vi "BPM.vi"() -> ()   [LabVIEW 2016]
uses:
  <vilib>/rvi/interface/nirviOpenFPGA/nirviOpenFPGA.xnode
  FPGA/BPM FPGA.vi
  <vilib>/rvi/interface/nirviReadWriteControl/nirviReadWriteControl.xnode
  <vilib>/Instr/_visa.llb/VISA Configure Serial Port (Instr).vi
  <vilib>/Utility/error.llb/Error Cluster From Error Code.vi
  <vilib>/rvi/errors/niLvFpgaAdjustHostInterfaceError.vi
  FPGA Bitfiles/Controlsoftware2_FPGATarget7_BPMFPGA_nBaxFvqMFXU.lvbitx
  <vilib>/FPGAPlugInAG/cRIO-9074/niLvFpga_Open_cRIO-9074.vi
  NiFpgaLv.dll
panel:
  out "einzel readbacks setpoints":fxp<+/-,26,5>[](array[numeric])
  out "einzel readbacks readbacks":fxp<+/-,26,5>[](array[numeric])
  out "chop index":i32
  out "element":string="0.00E+00\r\n"
  in  "source cage Ion gauge Cluster 4":T1
  out "source cage Ion gauge Cluster 2":T1={"beam line pressure  Gauge "="9.90E+09\r\n", "Turbo convectorn Gauge "="0.00E+00\r\n", "Steerer Convectro Gauge "="2.40E-08\r\n", "Ion gauge2"="7.60E-01\r\n"}
  out "read buffer":string="0.00E+00\r\n"
  out "error out":errorcluster
  out "BPM 2 x10":bool
  out "BPM 2":bool
  out "BPM 1 x10":bool
  out "BPM 1":bool
  # "0 run\n1 divert\n2 offset\n3 chop to detector"
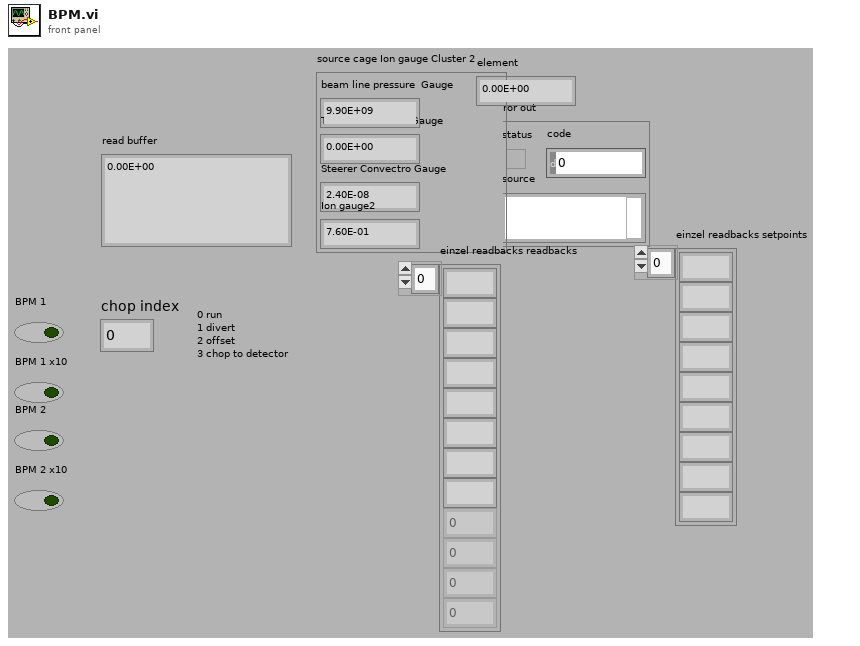
[diagram p1: front panel]
types:
  T1 = cluster{"beam line pressure  Gauge ":string, "Turbo convectorn Gauge ":string, "Steerer Convectro Gauge ":string, "Ion gauge2":string}
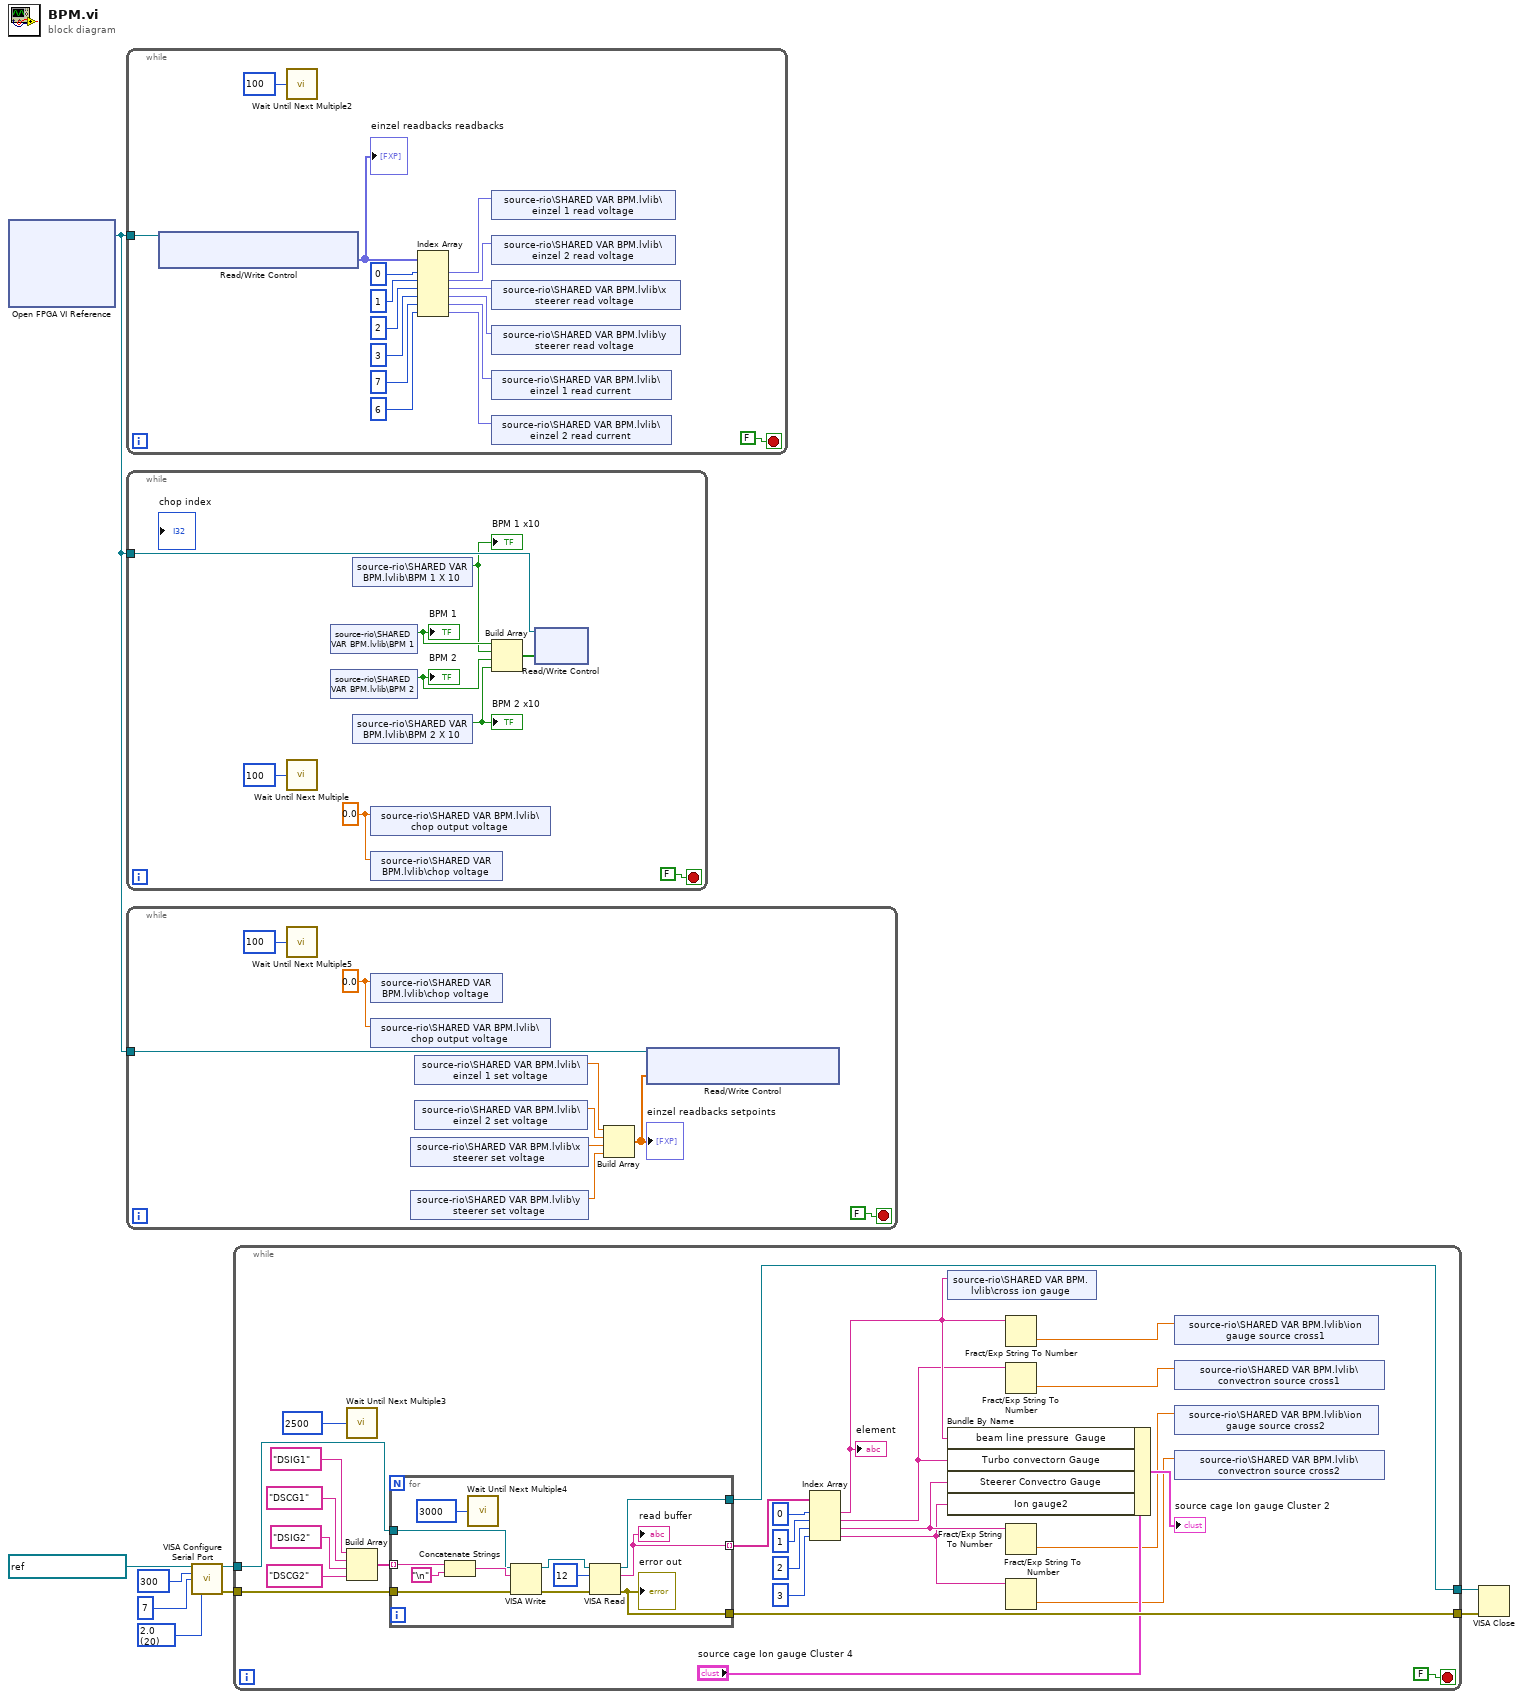
[diagram p0: block diagram]
diagram:
  w6 = u16 20 items=["1.0"=10, "1.5"=15, "2.0"=20] ("stop bits (10: 1 bit)")
  n1 = xnode "Open FPGA VI Reference"() -> ("FPGA VI Reference Out"=w1:refnum<k20>)  [unwired: 2 in, 1 out]
  n2 = while {
    tunnel: w1 -> [w25]
    stop <- FALSE stop-if-true
    n3 = xnode "Read/Write Control"("FPGA VI Reference In"=w25) -> ("einzel readbacks readbacks"=w22:fxp<+/-,26,5>[])  [unwired: 1 in, 2 out]
    "einzel readbacks readbacks" <- w22
    n4 = call "Wait Until Next Multiple2"("Count(mSec)"=u32 100) -> ()  [unwired: 1 out]
    n5 = Index Array(array=w22, index #1=0 ("index"), index #2=1 ("index"), index #3=2 ("index"), index #4=3 ("index"), index #5=7 ("index"), index #6=6 ("index")) -> (element #1=w10:fxp<+/-,26,5>, element #2=w11:fxp<+/-,26,5>, element #3=w15:fxp<+/-,26,5>, element #4=w14:fxp<+/-,26,5>, element #5=w13:fxp<+/-,26,5>, element #6=w12:fxp<+/-,26,5>)
    n6 = shared-variable "source-rio\\SHARED VAR BPM.lvlib\\einzel 1 read voltage"(w10) -> ()  [unwired: 1 in, 1 out]
    n7 = shared-variable "source-rio\\SHARED VAR BPM.lvlib\\einzel 2 read voltage"(w11) -> ()  [unwired: 1 in, 1 out]
    n8 = shared-variable "source-rio\\SHARED VAR BPM.lvlib\\x steerer read voltage"(w15) -> ()  [unwired: 1 in, 1 out]
    n9 = shared-variable "source-rio\\SHARED VAR BPM.lvlib\\y steerer read voltage"(w14) -> ()  [unwired: 1 in, 1 out]
    n10 = shared-variable "source-rio\\SHARED VAR BPM.lvlib\\einzel 1 read current"(w13) -> ()  [unwired: 1 in, 1 out]
    n11 = shared-variable "source-rio\\SHARED VAR BPM.lvlib\\einzel 2 read current"(w12) -> ()  [unwired: 1 in, 1 out]
  }
  n12 = while {
    tunnel: w1 -> [w34]
    stop <- FALSE stop-if-true
    w26 = 0.0 ("chop output voltage")
    n13 = call "Wait Until Next Multiple"("Count(mSec)"=u32 100) -> ()  [unwired: 1 out]
    n14 = shared-variable "source-rio\\SHARED VAR BPM.lvlib\\BPM 1"() -> (w33:bool)  [unwired: 1 in, 1 out]
    "BPM 1" <- w33
    n15 = shared-variable "source-rio\\SHARED VAR BPM.lvlib\\BPM 2"() -> (w31:bool)  [unwired: 1 in, 1 out]
    "BPM 2" <- w31
    n16 = shared-variable "source-rio\\SHARED VAR BPM.lvlib\\BPM 1 X 10"() -> (w32:bool)  [unwired: 1 in, 1 out]
    "BPM 1 x10" <- w32
    n17 = shared-variable "source-rio\\SHARED VAR BPM.lvlib\\BPM 2 X 10"() -> (w30:bool)  [unwired: 1 in, 1 out]
    "BPM 2 x10" <- w30
    n18 = shared-variable "source-rio\\SHARED VAR BPM.lvlib\\chop output voltage"(w26) -> ()  [unwired: 1 in, 1 out]
    n19 = shared-variable "source-rio\\SHARED VAR BPM.lvlib\\chop voltage"(w26) -> ()  [unwired: 1 in, 1 out]
    n20 = Build Array(w33, w32, w31, w30) -> (w29:bool[])
    n21 = xnode "Read/Write Control"("FPGA VI Reference In"=w34, "BPM"=w29) -> ()  [unwired: 1 in, 2 out]
  }
  n22 = while {
    tunnel: w1 -> [w40]
    stop <- FALSE stop-if-true
    w41 = 0.0 ("chop output voltage")
    n23 = call "Wait Until Next Multiple5"("Count(mSec)"=u32 100) -> ()  [unwired: 1 out]
    n24 = shared-variable "source-rio\\SHARED VAR BPM.lvlib\\chop voltage"(w41) -> ()  [unwired: 1 in, 1 out]
    n25 = shared-variable "source-rio\\SHARED VAR BPM.lvlib\\chop output voltage"(w41) -> ()  [unwired: 1 in, 1 out]
    n26 = shared-variable "source-rio\\SHARED VAR BPM.lvlib\\x steerer set voltage"() -> (w36:dbl)  [unwired: 1 in, 1 out]
    n27 = shared-variable "source-rio\\SHARED VAR BPM.lvlib\\y steerer set voltage"() -> (w35:dbl)  [unwired: 1 in, 1 out]
    n28 = shared-variable "source-rio\\SHARED VAR BPM.lvlib\\einzel 1 set voltage"() -> (w39:dbl)  [unwired: 1 in, 1 out]
    n29 = shared-variable "source-rio\\SHARED VAR BPM.lvlib\\einzel 2 set voltage"() -> (w38:dbl)  [unwired: 1 in, 1 out]
    n30 = Build Array(w39, w38, w36, w35) -> (w37:dbl[])
    "einzel readbacks setpoints" <- w37
    n31 = xnode "Read/Write Control"("FPGA VI Reference In"=w40, "einzel readbacks setpoints"=w37) -> ()  [unwired: 1 in, 2 out]
  }
  n32 = call-poly "VISA Configure Serial Port"("VISA resource name"=refnum<visa-resource-name> "ASRL1::INSTR", "baud rate (9600)"=u32 300, "data bits (8)"=u16 7, "stop bits (10: 1 bit)"=w6) -> ("VISA resource name out"=w5:refnum<visa-resource-name>, "error out"=w4:errorcluster)  [unwired: 10 in]
  n33 = while {
    tunnel: w5 -> [w66]
    tunnel: w4 -> [w65]
    tunnel: [w64] -> w3
    tunnel: [w63] -> w2
    stop <- FALSE stop-if-true
    n34 = call "Wait Until Next Multiple3"("Count(mSec)"=u32 2500) -> ()  [unwired: 1 out]
    n35 = Build Array("DSIG1" ("write buffer"), "DSCG1" ("write buffer"), "DSIG2" ("write buffer"), "DSCG2" ("write buffer")) -> (w67:string[])
    n36 = for {
      tunnel: w67 -> [w77] mode=indexing
      tunnel: w66 -> [w75]
      tunnel: w65 -> [w74]
      tunnel: [w73] -> w62 mode=indexing
      tunnel: [w72] -> w64
      tunnel: [w71] -> w63
      n37 = Concatenate Strings(w77, "\n") -> (w76:string)
      n38 = call "Wait Until Next Multiple4"("Count(mSec)"=u32 3000) -> ()  [unwired: 1 out]
      n39 = VISA Write(VISA resource name=w75, write buffer=w76, error in (no error)=w74) -> (VISA resource name out=w80:refnum<visa-resource-name>, error out=w79:errorcluster)  [unwired: 1 out]
      n40 = VISA Read(VISA resource name=w80, byte count=u32 12, error in (no error)=w79) -> (VISA resource name out=w71:refnum<visa-resource-name>, read buffer=w73:string, error out=w72:errorcluster)  [unwired: 1 out]
      "error out" <- w72
      "read buffer" <- w73
    }
    n41 = Index Array(array=w62, index #1=0 ("index"), index #2=1 ("index"), index #3=2 ("index"), index #4=3 ("index")) -> (element #1=w51:string, element #2=w50:string, element #3=w49:string, element #4=w48:string)
    "element" <- w51
    n42 = shared-variable "source-rio\\SHARED VAR BPM.lvlib\\cross ion gauge"(w51) -> ()  [unwired: 1 in, 1 out]
    n43 = Bundle By Name(cluster="source cage Ion gauge Cluster 4", "beam line pressure  Gauge"=w51, "Turbo convectorn Gauge"=w50, "Steerer Convectro Gauge"=w49, "Ion gauge2"=w48) -> (→"source cage Ion gauge Cluster 2":T1)
    n44 = Fract/Exp String To Number(string=w51) -> (number=w47:dbl)  [unwired: 3 in, 1 out]
    n45 = Fract/Exp String To Number(string=w50) -> (number=w45:dbl)  [unwired: 3 in, 1 out]
    n46 = Fract/Exp String To Number(string=w49) -> (number=w44:dbl)  [unwired: 3 in, 1 out]
    n47 = Fract/Exp String To Number(string=w48) -> (number=w46:dbl)  [unwired: 3 in, 1 out]
    n48 = shared-variable "source-rio\\SHARED VAR BPM.lvlib\\ion gauge source cross1"(w47) -> ()  [unwired: 1 in, 1 out]
    n49 = shared-variable "source-rio\\SHARED VAR BPM.lvlib\\convectron source cross1"(w45) -> ()  [unwired: 1 in, 1 out]
    n50 = shared-variable "source-rio\\SHARED VAR BPM.lvlib\\ion gauge source cross2"(w44) -> ()  [unwired: 1 in, 1 out]
    n51 = shared-variable "source-rio\\SHARED VAR BPM.lvlib\\convectron source cross2"(w46) -> ()  [unwired: 1 in, 1 out]
  }
  n52 = VISA Close(VISA resource name=w2, error in (no error)=w3) -> ()  [unwired: 1 out]
